vi "Module ID.vi"(11 "Messaging Client in":refnum<class "Messaging Server Client.lvclass">) -> (2 "Module ID":string)   [LabVIEW 2020, in "Volatus.lvlib" / "Messaging Server Client.lvclass"]
uses:
  Messaging Server Client.lvclass
  Messaging Server Client.lvclass/Messaging Server Client.ctl
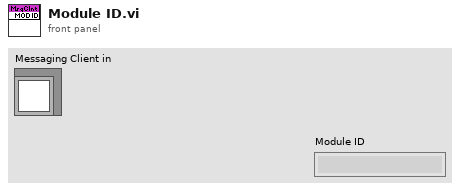
[diagram p1: front panel]
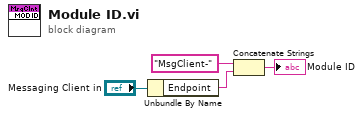
[diagram p0: block diagram]
diagram:
  n1 = Unbundle By Name("Messaging Client in") -> ("Endpoint"=w2:string)
  n2 = Concatenate Strings("MsgClient-", w2) -> (→"Module ID":string)
